vi "SpecAn Mode Set.vi"(0 "VISA In":refnum<visa-resource-name>, 5 "Error In":errorcluster, 6 "Mode (0: Swept SA)":i32(ring) items=["Swept SA", "Channel Power", "Occupied Bandwidth", "Power Stat CCDF", "Adjacent Channel Power", "Burst Power", "Spurious Emissions", "Spectrum Emission Mask", "List Sweep", "TOI", "Harmonic"]) -> (14 "VISA Out":refnum<visa-resource-name>, 19 "Error Out":errorcluster)   [LabVIEW 2015]
uses:
  Controls/FGV Action SpecAn Model.ctl
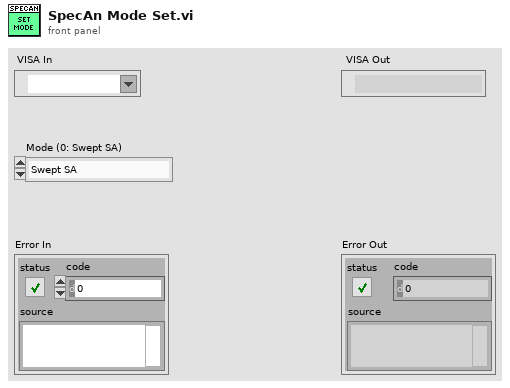
[diagram p1: front panel]
types:
  T1 = typedef "FGV Action SpecAn Model.ctl" = enum16{"Get", "Set"}
  T2 = typedef "SpecAn Model.ctl" = enum16{"E4440", "N9030"}
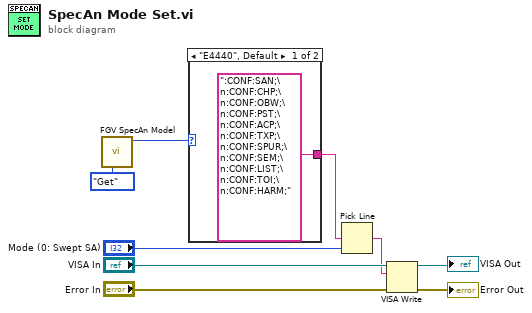
[diagram p0: block diagram]
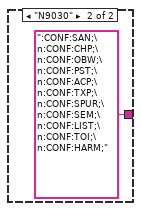
[diagram p2: hidden frame]
diagram:
  n1 = call "FGV SpecAn Model.vi"("Action"=FGV_Action_SpecAn_Model."Get") -> ("SA Model"=w1:T2)  [unwired: 6 in, 1 out]
  n2 = case shown="\"E4440\", Default" w1 {
    tunnel: [":CONF:SAN;\n:CONF:CHP;\n:CONF:OBW;\n:CONF:PST;\n:CONF:ACP;\n:CONF:TXP;\n:CONF:SPUR;\n:CONF:SEM;\n:CONF:LIST;\n:CONF:TOI;\n:CONF:HARM;" ":CONF:SAN;\n:CONF:CHP;\n:CONF:OBW;\n:CONF:PST;\n:CONF:ACP;\n:CONF:TXP;\n:CONF:SPUR;\n:CONF:SEM;\n:CONF:LIST;\n:CONF:TOI;\n:CONF:HARM;"] -> w5
    frame "E4440", Default {
    }
    frame "N9030" {
    }
  }
  n3 = Pick Line(multi-line string=w5, line index="Mode (0: Swept SA)") -> (output string=w3:string)  [unwired: 1 in]
  n4 = VISA Write(VISA resource name="VISA In", write buffer=w3, error in (no error)="Error In") -> (VISA resource name out=→"VISA Out":refnum<visa-resource-name>, error out=→"Error Out":errorcluster)  [unwired: 1 out]
